vi "SH_findBest.vi"(6 "Shapelets Num":i32=64, 7 "Fitness Values":dbl[](array[numeric]), 8 "ShapeletClass in":refnum<class "Shapelets Search Brute Force.lvclass">) -> (2 "Best Indicies":i32[](array[numeric]), 3 "ShapeletClass out":refnum<class "Shapelets Search Brute Force.lvclass">)   [LabVIEW 2016, in "Shapelets Search (Brute Force).lvlib" / "Shapelets Search Brute Force.lvclass"]
uses:
  Shapelets Search Brute Force.lvclass
panel:
  # "This VI is a part of BCI Design library, http://www.ru-bci.org \nCopyright © 2020, Sotnikov Peter, All rights reserved. License: GNU GPLv3"
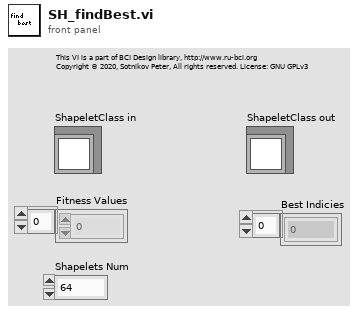
[diagram p1: front panel]
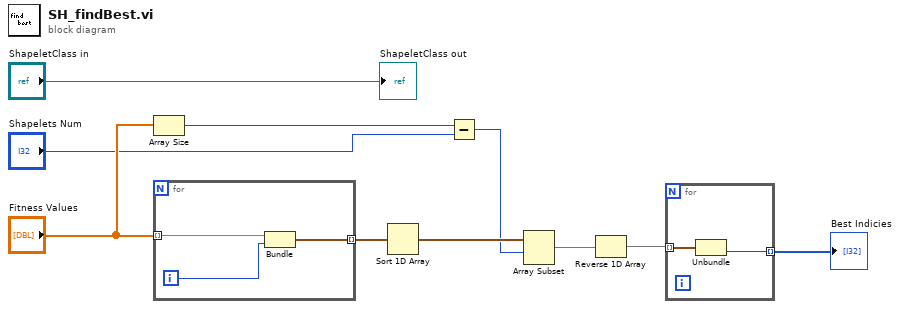
[diagram p0: block diagram]
diagram:
  n1 = Array Size(array="Fitness Values") -> (size(s)=w6:i32)
  n2 = for {
    tunnel: "Fitness Values" -> [w13] mode=indexing
    tunnel: [w11] -> w10 mode=indexing
    i -> [w12]
    n3 = Bundle("f"=w13, w12) -> (w11:cluster{"f":dbl, i32})  [unwired: 1 in]
  }
  n4 = Sort 1D Array(array=w10) -> (sorted array=w8:cluster{"f":dbl, i32}[])
  n5 = Subtract(x=w6, y="Shapelets Num") -> (x-y=w5:i32)
  n6 = Array Subset(array=w8, index=w5) -> (w2:cluster{"f":dbl, i32}[])  [unwired: 1 in]
  n7 = Reverse 1D Array(array=w2) -> (reversed array=w1:cluster{"f":dbl, i32}[])
  n8 = for {
    tunnel: w1 -> [w15] mode=indexing
    tunnel: [w14] -> w4 mode=indexing
    n9 = Unbundle(w15) -> (w14:i32)  [unwired: 1 out]
  }
  "Best Indicies" <- w4
  "ShapeletClass out" <- "ShapeletClass in"
